vi "SetSettings.vi"(8 "error in (no error)":errorcluster, 10 "Variant":variant, 11 "NHRDCPowerModel in":refnum<class "NHRDCPowerModel.lvclass">) -> (0 "error out":errorcluster, 3 "NHRDCPowerModel Out":refnum<class "NHRDCPowerModel.lvclass">)   [LabVIEW 2018, in "AcPwrPlugins.lvlib" / "NHRDCPowerModel.lvclass"]
doc: "This VI sets the instruments properties."
uses:
  NHRDCPowerModel.lvclass
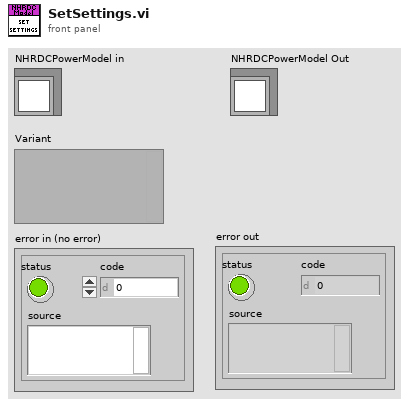
[diagram p1: front panel]
types:
  T1 = typedef "AcPwrPlugins.lvlib/NHRDCPower.lvclass/Measurements.ctl" = cluster{"Handle":string, "Name":string, "Enabled":bool, "Measurement Value":sgl, "Measurement Type":enum16{"Power", "Current", "Voltage"}}[]
  T2 = typedef "AcPwrPlugins.lvlib/NHRDCPower.lvclass/Device(s)Settings.ctl" = cluster{"MeasName":string, "Modules":T3}
  T3 = typedef "AcPwrPlugins.lvlib/NHRDCPower.lvclass/Modules.ctl" = cluster{"Handle":string, "Name":string, "id query (Yes)":bool, "reset device (Yes)":bool, "Connected":bool, "Initial Battery Detect Voltage (0)":dbl, "SafetySettings":cluster{"SetWatchDog?":bool, "Voltage (V)":dbl, "Current (A)":dbl, "Power (W)":dbl, "Voltage Delay (s)":dbl, "Current Delay (s)":dbl, "Power Delay (s)":dbl}, "Options String":string, "Aperture Time (s)":dbl, "operating state (Off)":i32, "OutputSettings":cluster{"Voltage (V)":dbl, "Current (A)":dbl, "Resistance (Ohms)":dbl, "Power (W)":dbl, "Enable Voltage":bool, "Enable Current":bool, "Enable Resistance":bool, "Enable Power":bool, "Macro After Step Delay  (s)":dbl, "Wait Value (V, A, W)":dbl, "Enable Wait":bool, "Wait on Value":i32}, "SlewRate":cluster{"Set Voltage Rate V/S":dbl, "Set Current Rate A/S":dbl, "Set Resistance Rate R/S":dbl, "Set Power Rate W/S":dbl}, "Macro":cluster{"Save Macro?":bool, "Load Macro From File?":bool, "Run Macro Continuously?":bool, "Use Macros?":bool, "Load Macro File Path":path, "Save Macro File Path":string}, "Regulation Gain (1=100%)":dbl, "UpdatingOntheFly":bool}[]
  T4 = typedef "AcPwrShared.lvlib/Database Settings.ctl" = cluster{"Data Source":string, "ICDAS to Model Table":string, "Model to ICDAS Table":string}
  T5 = cluster{"Device(s)Settings":T2, "Database Settings":T4}
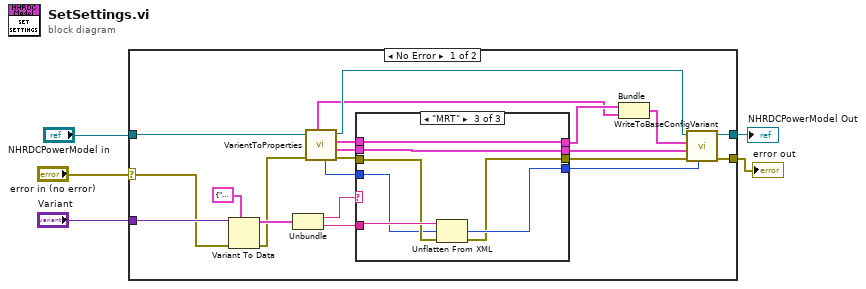
[diagram p0: block diagram]
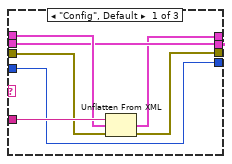
[diagram p2: hidden frame]
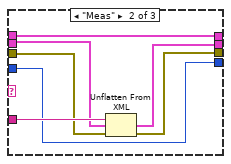
[diagram p3: hidden frame]
diagram:
  n1 = case shown="No Error" "error in (no error)" {
    selector: "error in (no error)" -> [w25 w49]
    tunnel: [w14 w49] -> w1
    tunnel: "NHRDCPowerModel in" -> [w20 w48]
    tunnel: "Variant" -> [w26 _]
    tunnel: [w13 w48] -> w2
    frame No Error {
      n2 = Variant To Data(error in=w25, type=cluster{string, string} {"", ""}, Variant=w26) -> (data=w23:cluster{string, string}, error out=w19:errorcluster)
      n3 = Unbundle(w23) -> (w21:string, w22:string)
      n4 = call "VarientToProperties.vi"("error in (no error)"=w19, "AcPwrPlugins.lvlib:NHRDCModel.lvclass"=w20) -> ("error out"=w16:errorcluster, "Measurements"=w17:T1, "Device(s)Settings"=w18:T2, "AcPwrPlugins.lvlib:NHRDCModel.lvclass"=w11:refnum<class "NHRDCPowerModel.lvclass">, "Measurement Refresh Time (ms)"=w15:u32, "Database Settings"=w7:T4)  [unwired: 4 in]
      n5 = case shown="\"MRT\"" w21 {
        tunnel: [w27 w34 w45] -> w10
        tunnel: w16 -> [w31 w36 w42]
        tunnel: w22 -> [w33 w40 w47]
        tunnel: w18 -> [w32 w39 w44]
        tunnel: w17 -> [w29 w38 w43]
        tunnel: w15 -> [w30 w37 w41]
        tunnel: [w28 w39 w44] -> w8
        tunnel: [w29 w35 w43] -> w9
        tunnel: [w30 w37 w46] -> w12
        frame "Config", Default {
          n6 = Unflatten From XML(xml string=w33, type=w32, error in (no error)=w31) -> (value=w28:T2, error out=w27:errorcluster)
        }
        frame "Meas" {
          n7 = Unflatten From XML(xml string=w40, type=w38, error in (no error)=w36) -> (value=w35:T1, error out=w34:errorcluster)
        }
        frame "MRT" {
          n8 = Unflatten From XML(xml string=w47, type=w41, error in (no error)=w42) -> (value=w46:u32, error out=w45:errorcluster)
        }
      }
      n9 = Bundle("Device(s)Settings"=w8, "Database Settings"=w7) -> (w6:T5)  [unwired: 1 in]
      n10 = call-dynamic "WriteToBaseConfigVariant.vi"("Measurement Refresh Time (ms)"=w12, "error in (no error)"=w10, "Meas"=w9, "Config"=w6, "NHRDCModel in"=w11) -> ("error out"=w14:errorcluster, "NHRDCModel out"=w13:refnum<class "NHRDCPowerModel.lvclass">)  [unwired: 5 in]
    }
    frame Error {
    }
  }
  "error out" <- w1
  "NHRDCPowerModel Out" <- w2
